vi "Read Network Master.vi"(8 "error in (no error)":errorcluster, 11 "Serial in":refnum<class "Serial.lvclass">) -> (0 "error out":errorcluster, 2 "Network Master":refnum<class "Network Master.lvclass">, 3 "Serial out":refnum<class "Serial.lvclass">)   [LabVIEW 2021, in "Serial.lvclass"]
uses:
  Serial.lvclass
  C:/my_projects/projects/Algorithms/Labview/21/Master CR/Master CR.lvclass
  Modbus_v121c/Network Protocol/Network Master/Network Master.lvclass
  Master CR.lvclass/Master CR.ctl
  Master CR.lvclass
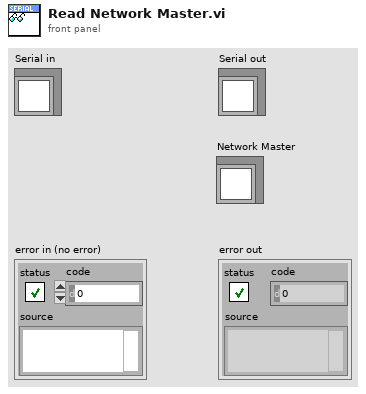
[diagram p1: front panel]
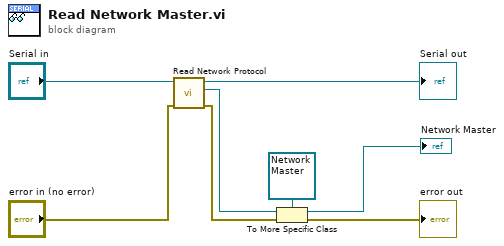
[diagram p0: block diagram]
diagram:
  n1 = call "Read Network Protocol.vi"("error in (no error)"="error in (no error)", "Master CR in"="Serial in") -> ("error out"=w5:errorcluster, "Network Protocol"=w2:refnum<class "Network Protocol.lvclass">, "Master CR out"=→"Serial out":refnum<class "Serial.lvclass">)  [unwired: 7 in]
  n2 = To More Specific Class(target class=refnum<class "Network Master.lvclass"> refnum ("Network Master"), reference=w2, error in=w5) -> (specific class reference=→"Network Master":refnum<class "Network Master.lvclass">, error out=→"error out":errorcluster)
